vi "UsrProfiles-Copy current-create new.vi"(8 "error in (no error)":errorcluster, 11 "New profile's filepath":path) -> (0 "error out":errorcluster)   [LabVIEW 2020]
uses:
  Typedefs/Save-Load enum.ctl
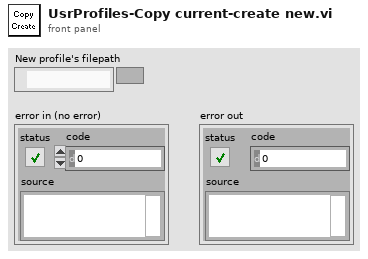
[diagram p1: front panel]
types:
  T1 = typedef "Save-Load enum.ctl" = enum16{"Save to file", "Load from file", "Compare from file", "Save Backup"}
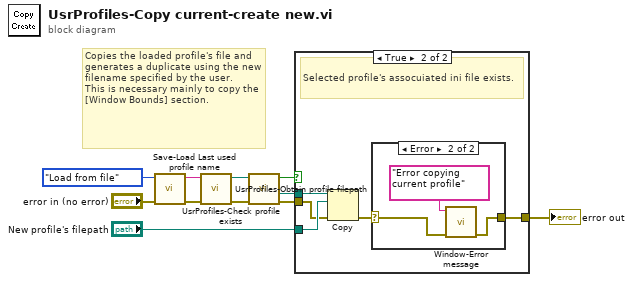
[diagram p0: block diagram]
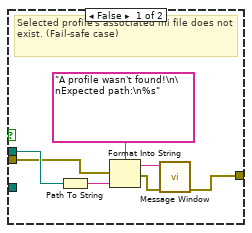
[diagram p2: hidden frame]
diagram:
  # "Copies the loaded profile's file and generates a duplicate using the new filename specified by the user.\nThis is necessary mainly to copy the [Window Bounds] section."
  n1 = call "Save-Load Last used profile name.vi"("error in"="error in (no error)", "Function"=Save-Load_enum."Load from file") -> ("error out"=w1:errorcluster, "Last used profile for selected user"=w9:string)  [unwired: 7 in, 1 out]
  n2 = call "UsrProfiles-Obtain profile filepath.vi"("error in"=w1, "Profile name"=w9) -> ("error out"=w3:errorcluster, "Profile filepath"=w2:path)  [unwired: 8 in]
  n3 = call "UsrProfiles-Check profile exists.vi"("error in"=w3, "Profile file path"=w2) -> ("error out"=w4:errorcluster, "Profile's file path"=w5:path, "Profile file exists"=w6:bool)  [unwired: 7 in]
  n4 = case shown="True" w6 {
    tunnel: w4 -> [w14 w20]
    tunnel: w5 -> [w18 w23]
    tunnel: "New profile's filepath" -> [_ w22]
    tunnel: [w12 w21] -> w11
    frame False {
      # "Selected profile's associated ini file does not exist. (Fail-safe case)"
      n5 = Path To String(path=w18) -> (string=w17:string)
      n6 = Format Into String(format string="A profile wasn't found!\n\nExpected path:\n%s", error in=w14, w17) -> (resulting string=w15:string, error out=w13:errorcluster)  [unwired: 1 in]
      n7 = call "Message Window.vi"("error in (no error)"=w13, "Message string"=w15) -> ("error out (no error)"=w12:errorcluster)  [unwired: 9 in]
    }
    frame True {
      # "Selected profile's assocuiated ini file exists."
      n8 = Copy(8:w20, 10:w22, 11:w23) -> (0:w19:errorcluster)  [unwired: 2 in, 2 out]
      n9 = case shown="Error" w19 {
        selector: w19 -> [w24 w26]
        tunnel: [w24 w25] -> w21
        frame No Error {
        }
        frame Error {
          n10 = call "Window-Error message.vi"("error in (no error)"=w26, "Message"="Error copying current profile") -> ("Error Out (no error)"=w25:errorcluster)  [unwired: 9 in]
        }
      }
    }
  }
  "error out" <- w11
